vi "_API_BINANCE_POST_NewOrder.vi"(0 "BinanceAPI in":refnum<class "BinanceAPI_.lvclass">, 5 "NewOrder":T1={"symbol"="CAKEUSDT", "side"=enum."SELL", "type"=enum."MARKET", "timeInForce"=enum."NaN", "quantity"=0.60000000000000000002, "quoteOrderQty"=nan, "price"=nan, "newClientOrderId"="NaN", "stopPrice"=nan, "icebergQty"=nan, "newOrderRespType"=enum."NaN", "recvWindow"=5000, "timestamp"=0}, 11 "error in (no error)":errorcluster) -> (4 "BinanceAPI out":refnum<class "BinanceAPI_.lvclass">, 14 "Body":string, 15 "error out":errorcluster)   [LabVIEW 2022 SP3, in "BinanceAPI_.lvclass"]
doc: "https://binance-docs.github.io/apidocs/spot/en/#new-order-trade"
uses:
  BinanceAPI_.lvclass
  BinanceAPI_.lvclass/BinanceAPI_.ctl
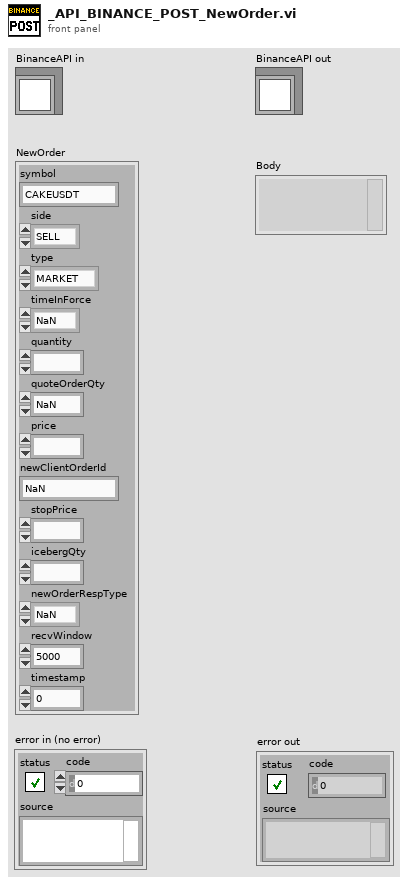
[diagram p1: front panel]
types:
  T1 = cluster{"symbol":string, "side":enum16{"NaN", "SELL", "BUY"}, "type":enum16{"NaN", "LIMIT", "MARKET", "STOP_LOSS", "STOP_LOSS_LIMIT", "TAKE_PROFIT", "TAKE_PROFIT_LIMIT", "LIMIT_MAKER"}, "timeInForce":enum16{"NaN", "GTC", "IOC", "FOK"}, "quantity":ext, "quoteOrderQty":dbl, "price":ext, "newClientOrderId":string, "stopPrice":ext, "icebergQty":ext, "newOrderRespType":enum16{"NaN", "ACK", "RESULT", "FULL"}, "recvWindow":i32, "timestamp":i32}
  T2 = enum16{"SPOT", "USDT_FUTURES", "COIN_FUTURES", "VANILLA"}
  T3 = enum16{"NaN", "LIMIT", "MARKET", "STOP_LOSS", "STOP_LOSS_LIMIT", "TAKE_PROFIT", "TAKE_PROFIT_LIMIT", "LIMIT_MAKER"}
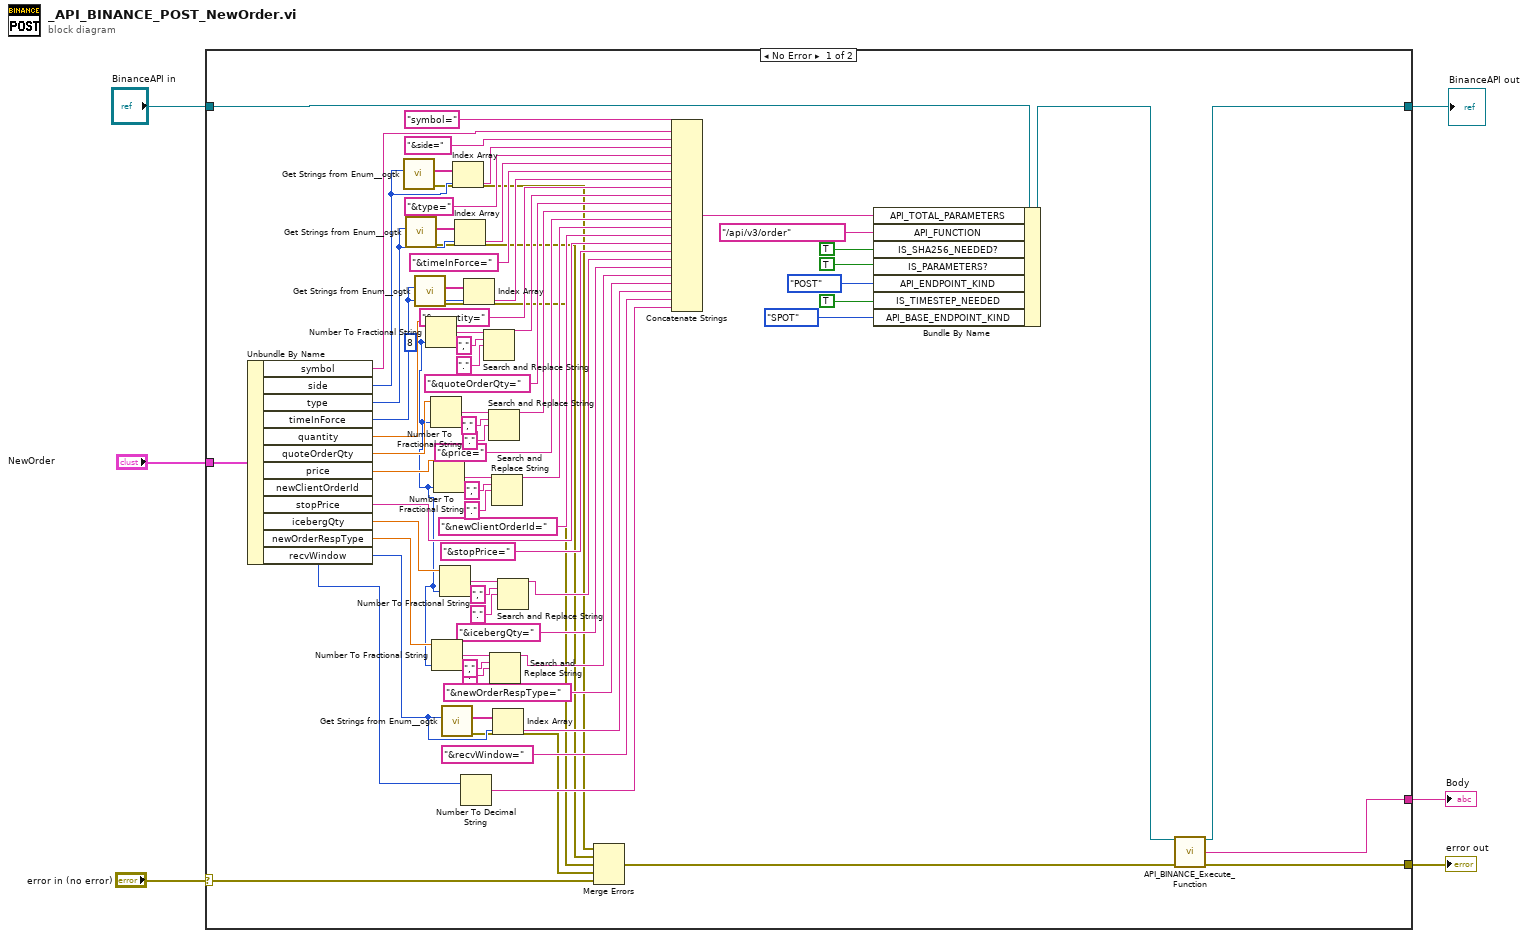
[diagram p0: block diagram]
diagram:
  n1 = case shown="No Error" "error in (no error)" {
    selector: "error in (no error)" -> [w34 w81]
    tunnel: [w9 w81] -> w5
    tunnel: [w11 w80] -> w1
    tunnel: "BinanceAPI in" -> [w35 w80]
    tunnel: "NewOrder" -> [w76 _]
    tunnel: [w7 _] -> w3
    frame No Error {
      w14 = i16 8 ("precision (6)")
      n2 = Unbundle By Name(w76) -> ("symbol"=w71:string, "side"=w50:enum16{"NaN", "SELL", "BUY"}, "type"=w49:T3, "timeInForce"=w48:enum16{"NaN", "GTC", "IOC", "FOK"}, "quantity"=w42:ext, "quoteOrderQty"=w37:dbl, "price"=w31:ext, "newClientOrderId"=w58:string, "stopPrice"=w27:ext, "icebergQty"=w23:ext, "newOrderRespType"=w47:enum16{"NaN", "ACK", "RESULT", "FULL"}, "recvWindow"=w52:i32)
      n3 = call <userlib>:"Get Strings from Enum__ogtk.vi"("Enum"=w50) -> ("error out"=w18:errorcluster, "Enum Strings"=w74:string[])  [unwired: 7 in, 2 out]
      n4 = call <userlib>:"Get Strings from Enum__ogtk.vi"("Enum"=w49) -> ("error out"=w19:errorcluster, "Enum Strings"=w68:string[])  [unwired: 7 in, 2 out]
      n5 = call <userlib>:"Get Strings from Enum__ogtk.vi"("Enum"=w48) -> ("error out"=w20:errorcluster, "Enum Strings"=w64:string[])  [unwired: 7 in, 2 out]
      n6 = Number To Fractional String(number=w42, precision (6)=w14) -> (F-format string=w46:string)  [unwired: 2 in]
      n7 = Number To Fractional String(number=w37, precision (6)=w14) -> (F-format string=w38:string)  [unwired: 2 in]
      n8 = Number To Fractional String(number=w23, precision (6)=w14) -> (F-format string=w25:string)  [unwired: 2 in]
      n9 = Number To Fractional String(number=w31, precision (6)=w14) -> (F-format string=w33:string)  [unwired: 2 in]
      n10 = Number To Fractional String(number=w27, precision (6)=w14) -> (F-format string=w28:string)  [unwired: 2 in]
      n11 = call <userlib>:"Get Strings from Enum__ogtk.vi"("Enum"=w47) -> ("error out"=w21:errorcluster, "Enum Strings"=w75:string[])  [unwired: 7 in, 2 out]
      n12 = Index Array(array=w74, index=w50) -> (element=w69:string)
      n13 = Index Array(array=w68, index=w49) -> (element=w66:string)
      n14 = Number To Decimal String(number=w52) -> (decimal integer string=w51:string)  [unwired: 1 in]
      n15 = Index Array(array=w64, index=w48) -> (element=w63:string)
      n16 = Search and Replace String(input string=w46, search string=",", replace string="." ("replace string (\"\")")) -> (result string=w43:string)  [unwired: 5 in, 3 out]
      n17 = Search and Replace String(input string=w38, search string=",", replace string="." ("replace string (\"\")")) -> (result string=w36:string)  [unwired: 5 in, 3 out]
      n18 = Search and Replace String(input string=w25, search string=",", replace string="." ("replace string (\"\")")) -> (result string=w22:string)  [unwired: 5 in, 3 out]
      n19 = Search and Replace String(input string=w33, search string=",", replace string="." ("replace string (\"\")")) -> (result string=w30:string)  [unwired: 5 in, 3 out]
      n20 = Index Array(array=w75, index=w47) -> (element=w54:string)
      n21 = Search and Replace String(input string=w28, search string=",", replace string="." ("replace string (\"\")")) -> (result string=w26:string)  [unwired: 5 in, 3 out]
      n22 = Merge Errors(w18, w19, w20, w21, w34) -> (w10:errorcluster)
      n23 = Concatenate Strings("symbol=" ("Symbol"), w71, "&side=" ("Symbol"), w69, "&type=" ("Symbol"), w66, "&timeInForce=" ("Symbol"), w63, "&quantity=" ("Symbol"), w43, "&quoteOrderQty=" ("Symbol"), w36, "&price=" ("Symbol"), w30, "&newClientOrderId=" ("Symbol"), w58, "&stopPrice=" ("Symbol"), w26, "&icebergQty=" ("Symbol"), w22, "&newOrderRespType=" ("Symbol"), w54, "&recvWindow=" ("Symbol"), w51) -> (w73:string)
      n24 = Bundle By Name(cluster=w35, "API_TOTAL_PARAMETERS"=w73, "API_FUNCTION"="/api/v3/order", "IS_SHA256_NEEDED?"=TRUE, "IS_PARAMETERS?"=TRUE, "API_ENDPOINT_KIND"=enum16{"POST", "DELETE", "GET", "PUT"}."POST", "IS_TIMESTEP_NEEDED"=TRUE ("IS_PARAMETERS?"), "API_BASE_ENDPOINT_KIND"=T2."SPOT") -> (w12:refnum<class "BinanceAPI_.lvclass">)
      n25 = call "API_BINANCE_Execute_Function.vi"("BinanceAPI in"=w12, "error in (no error)"=w10) -> ("BinanceAPI out"=w11:refnum<class "BinanceAPI_.lvclass">, "Body"=w7:string, "error out"=w9:errorcluster)  [unwired: 9 in, 2 out]
    }
    frame Error {
    }
  }
  "error out" <- w5
  "Body" <- w3
  "BinanceAPI out" <- w1
